vi "Transform To Intensity.vi"(0 "PolarizationProcessor reference":refnum<k24>, 1 "imageOriginX_pixels":i32, 2 "imageOriginY_pixels":i32, 3 "sensorPolarPhase":i32(ring) items=["PolarPhase0", "PolarPhase45", "PolarPhase90", "PolarPhase135"], 5 "inputImage":u16[](array[numeric]), 7 "inputImageBitDepth":i32, 9 "outputMaxValue":u16, 11 "error in (no error)":errorcluster, 12 "imageWidth_pixels":i32, 13 "imageHeight_pixels":i32, 14 "Intensity buffer input":u16[](array[numeric])) -> (4 "PolarizationProcessor reference out":refnum<k24>, 6 "Intensity out":u16[](array[numeric]), 15 "error out":errorcluster)   [LabVIEW 2015]
uses:
  C:/code/Host/Installer/Scientific Camera Interfaces/LabVIEW/32_bit/Library_X86/Thorlabs.TSI.PolarizationInterfaces.dll
  code/Host/Installer/Scientific Camera Interfaces/LabVIEW/32_bit/Library_X86/Thorlabs.TSI.PolarizationInterfaces.dll
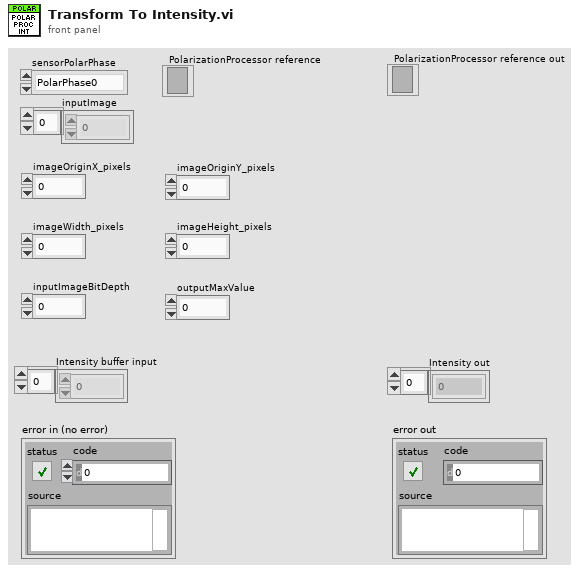
[diagram p1: front panel]
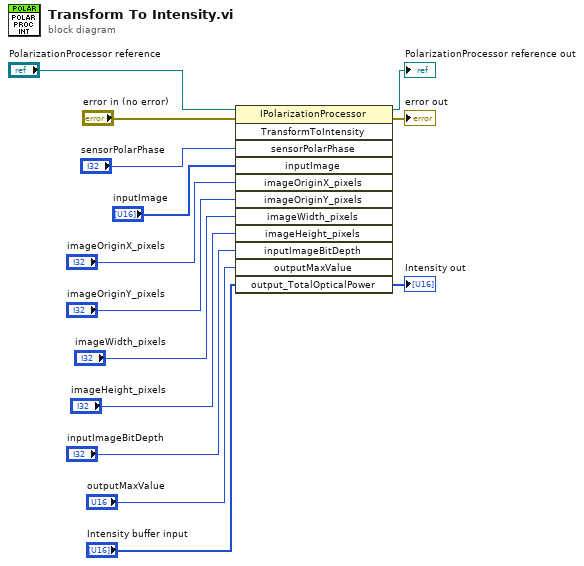
[diagram p0: block diagram]
diagram:
  n1 = invoke class="IPolarizationProcessor" method="TransformToIntensity"(reference="PolarizationProcessor reference", error in="error in (no error)", "sensorPolarPhase"="sensorPolarPhase", "inputImage"="inputImage", "imageOriginX_pixels"="imageOriginX_pixels", "imageOriginY_pixels"="imageOriginY_pixels", "imageWidth_pixels"="imageWidth_pixels", "imageHeight_pixels"="imageHeight_pixels", "inputImageBitDepth"="inputImageBitDepth", "outputMaxValue"="outputMaxValue", "output_TotalOpticalPower"="Intensity buffer input") -> (reference out=→"PolarizationProcessor reference out":refnum<k24>, error out=→"error out":errorcluster, "output_TotalOpticalPower"=→"Intensity out":u16[])  [unwired: 1 in, 9 out]
